vi "KE622x -- Set Math Mode Params.vi"(0 "Resource In":refnum<visa-resource-name>, 1 "Check For SCPI Errors? (T)":bool=TRUE, 7 "Math Mode Params In":T1={"Math Enabled?"=FALSE, "Math Mode"=enum."mX + b", "Slope (m)"=1.0, "Intercept (b)"=0.0} {"Intercept (b)" min=-9.99999e+20 max=9.99999e+20 format="%.5e"; "Slope (m)" min=-9.99999e+20 max=9.99999e+20 format="%.5e"}, 11 "error in (no error)":errorcluster, 12 "Read Back Set Values? (T)":bool=TRUE) -> (4 "Resource Out (dupl)":refnum<visa-resource-name>, 8 "Math Mode Params Out":T1={"Math Enabled?"=FALSE, "Math Mode"=enum."mX + b", "Slope (m)"=1.0, "Intercept (b)"=0.0} {"Intercept (b)" min=-9.99999e+20 max=9.99999e+20 format="%.5e"; "Slope (m)" min=-9.99999e+20 max=9.99999e+20 format="%.5e"}, 15 "error out":errorcluster)   [LabVIEW 2019, in "Keithley 622x.lvlib"]
doc: "Sets up and optionally enables math mode for measurements returned from the 2182/2182A nano-voltmeter."
uses:
  Keithley 622x.lvlib
  Typedefs/KE622x -- Math Mode Params.ctl
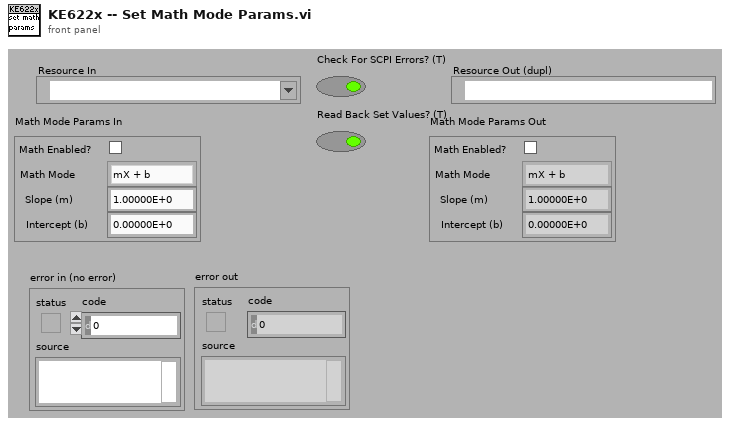
[diagram p1: front panel]
types:
  T1 = typedef "Keithley 622x.lvlib/KE622x -- Math Mode Params.ctl" = cluster{"Math Enabled?":bool, "Math Mode":enum16{"None", "mX + b", "m/X + b"}, "Slope (m)":dbl, "Intercept (b)":dbl}
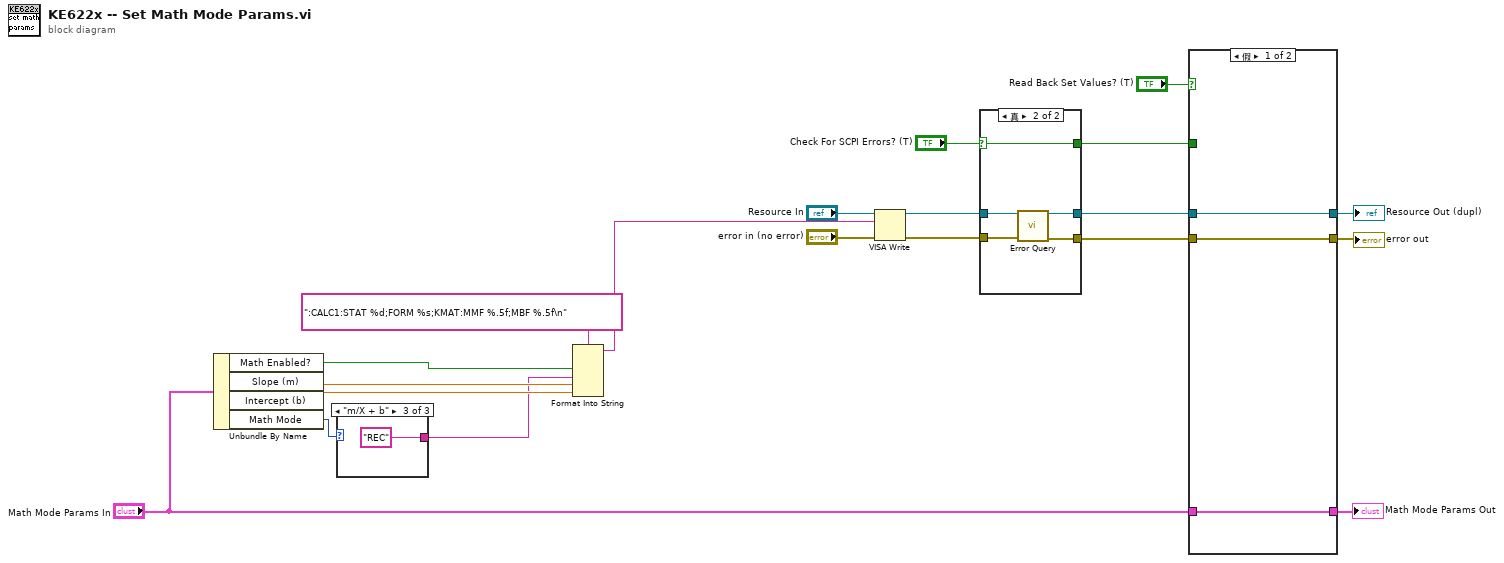
[diagram p0: block diagram]
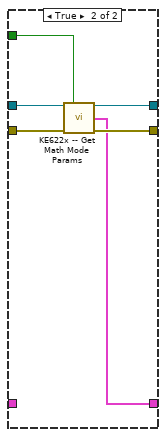
[diagram p2: hidden frame]
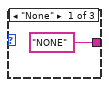
[diagram p3: hidden frame]
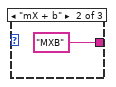
[diagram p4: hidden frame]
diagram:
  n1 = Unbundle By Name("Math Mode Params In") -> ("Math Enabled?"=w14:bool, "Slope (m)"=w12:dbl, "Intercept (b)"=w11:dbl, "Math Mode"=w10:enum16{"None", "mX + b", "m/X + b"})
  n2 = case shown="\"m/X + b\"" w10 {
    tunnel: ["NONE" "MXB" "REC"] -> w9
    frame "None" {
    }
    frame "mX + b" {
    }
    frame "m/X + b" {
    }
  }
  n3 = Format Into String(format string=":CALC1:STAT %d;FORM %s;KMAT:MMF %.5f;MBF %.5f\n", w14, w9, w12, w11) -> (resulting string=w13:string)  [unwired: 2 in, 1 out]
  n4 = VISA Write(VISA resource name="Resource In", write buffer=w13, error in (no error)="error in (no error)") -> (VISA resource name out=w17:refnum<visa-resource-name>, error out=w16:errorcluster)  [unwired: 1 out]
  n5 = case shown="真" "Check For SCPI Errors? (T)" {
    selector: "Check For SCPI Errors? (T)" -> [w24 w27]
    tunnel: w17 -> [w26 w31]
    tunnel: w16 -> [w25 w30]
    tunnel: [w25 w29] -> w5
    tunnel: [w26 w28] -> w6
    tunnel: [w24 w27] -> w4
    frame False {
    }
    frame True {
      n6 = call "Error Query.vi"("VISA Resource In"=w31, "error in (no error)"=w30) -> ("VISA Resource Out (dupl)"=w28:refnum<visa-resource-name>, "error out"=w29:errorcluster)  [unwired: 10 in, 2 out]
    }
  }
  n7 = case shown="假" "Read Back Set Values? (T)" {
    tunnel: "Math Mode Params In" -> [w34 _]
    tunnel: [w34 w35] -> w1
    tunnel: w6 -> [w33 w40]
    tunnel: w5 -> [w32 w39]
    tunnel: w4 -> [_ w38]
    tunnel: [w32 w37] -> w2
    tunnel: [w33 w36] -> w3
    frame False {
    }
    frame True {
      n8 = call "KE622x -- Get Math Mode Params.vi"("Resource In"=w40, "Check For SCPI Errors? (T)"=w38, "error in (no error)"=w39) -> ("Resource Out (dupl)"=w36:refnum<visa-resource-name>, "Math Mode Params"=w35:T1, "error out"=w37:errorcluster)  [unwired: 10 in]
    }
  }
  "Resource Out (dupl)" <- w3
  "error out" <- w2
  "Math Mode Params Out" <- w1
